vi "Configure Output.vi"(0 "VISA resource name":refnum<visa-resource-name>, 5 "Source Level (0)":dbl, 7 "Source Mode  (0: Voltage)":u16(ring) items=["Voltage", "Current"], 9 "Source Limit Level (0.1)":dbl=0.1, 11 "error in (no error)":errorcluster) -> (4 "VISA resource name out":refnum<visa-resource-name>, 15 "error out":errorcluster)   [LabVIEW 2025, in "Keithley 2450.lvlib"]
doc: "Configures whether the output is in terms of current or voltage, the amplitude of the output, and compliance settings."
uses:
  Keithley 2450.lvlib
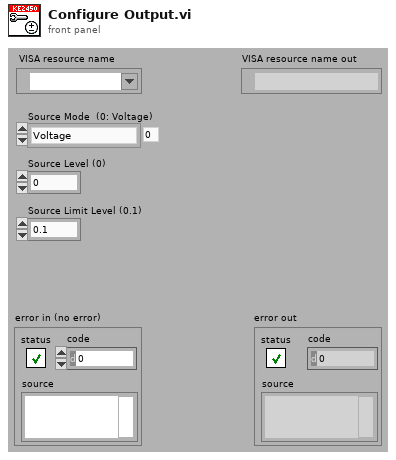
[diagram p1: front panel]
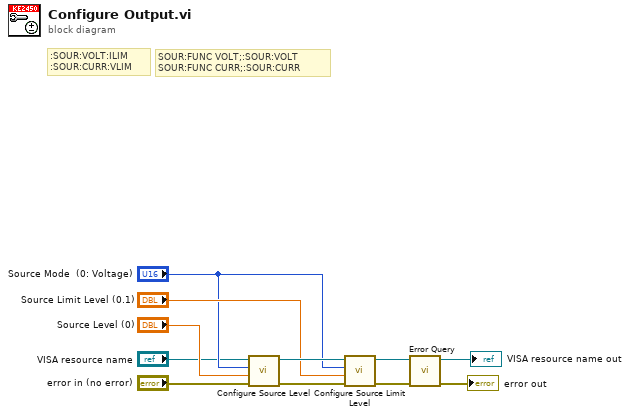
[diagram p0: block diagram]
diagram:
  # "SOUR:FUNC VOLT;:SOUR:VOLT\nSOUR:FUNC CURR;:SOUR:CURR"
  # ":SOUR:VOLT:ILIM\n:SOUR:CURR:VLIM"
  n1 = call "Configure Source Level.vi"("error in (no error)"="error in (no error)", "Source Level (1.0)"="Source Level (0)", "Function (0: Volts)"="Source Mode  (0: Voltage)", "VISA resource name"="VISA resource name") -> ("error out"=w9:errorcluster, "VISA resource name out"=w8:refnum<visa-resource-name>)  [unwired: 6 in]
  n2 = call "Configure Source Limit Level.vi"("error in (no error)"=w9, "Source Limit (1.0)"="Source Limit Level (0.1)", "Function (0: Volts)"="Source Mode  (0: Voltage)", "VISA resource name"=w8) -> ("error out"=w6:errorcluster, "VISA resource name out"=w7:refnum<visa-resource-name>)  [unwired: 6 in]
  n3 = call "Error Query.vi"("error in (no error)"=w6, "VISA resource name"=w7) -> ("error out"=→"error out":errorcluster, "VISA resource name out"=→"VISA resource name out":refnum<visa-resource-name>)  [unwired: 8 out]
